vi "query_cmd_single.vi"(6 "Parameter":variant, 7 "Command group":T3(ring), 8 "error in (no error)":errorcluster, 9 "Command ID":u8, 10 "Command subgroup":T2(ring), 11 "VISA resource name":refnum<visa-resource-name>) -> (0 "error out":errorcluster, 1 "formatted response":string, 2 "command packet":string, 3 "VISA resource name out":refnum<visa-resource-name>, 4 "response packet cluster":T1)   [LabVIEW 2018]
doc: "Query a command supported by the IC6 and format the response accordingly."
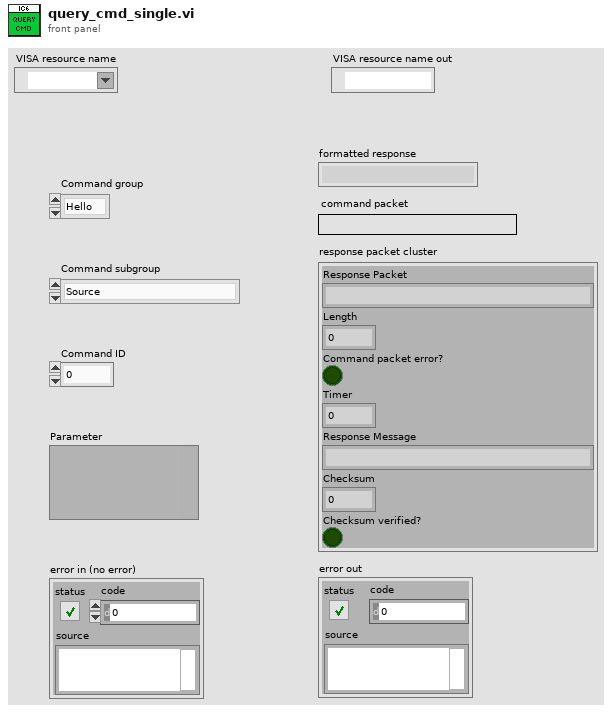
[diagram p1: front panel]
types:
  T1 = cluster{"Response Packet":string, "Length":u16, "Command packet error?":bool, "Timer":u8, "Response Message":string, "Checksum":u8, "Checksum verified?":bool}
  T2 = enum16{"Source", "General", "Input name", "Process name", "Logic", "Material", "Material name", "Output name", "Process", "Sensor", "Output type", "User message", "Layer", ""}
  T3 = enum16{"Hello", "Query", "Remote action", "Status", "Update"}
  T4 = enum16{"big-endian, network order", "native, host order", "little-endian"}
  T5 = enum16{"Crystal Fail", "Max Power", "Test", "A TEST", "R Lock", "L Lock", "Min Power", "Crystal Switch", "Crystal Sw Fail", "Carousel Open", "Control Delay", "Transfer Delay", "RateWatcher Delay", "RateWatcher Hold", "RateWatcher Sample", "Soak Hold Pre Con", "Soak Hold 1", "Soak Hold 2", "Abbr Average", "No or Neg. Average", "Time Pwr Complete", "Clock Hold", "End of Process", "CoDep Not Calibr", "One Layer Tagged", "Layers Tagged", "Too Many Layers", "Source Conflict", "Recorder Conflict", "Unable to Auto-Z", "DAC Error", "Testing XIU", "Backup Sensor", "Backup Delay"}
  T6 = cluster{"statement #":u8, "statement (hex string)":string}
  T7 = cluster{"Process number":u8, "Layer number":u8, "Parameter":i32}
  T8 = cluster{"Process number":u8, "Layer number":u8, "Parameter":dbl}
  T9 = cluster{"Process number":u8, "Layer number":u8, "Parameter":bool}
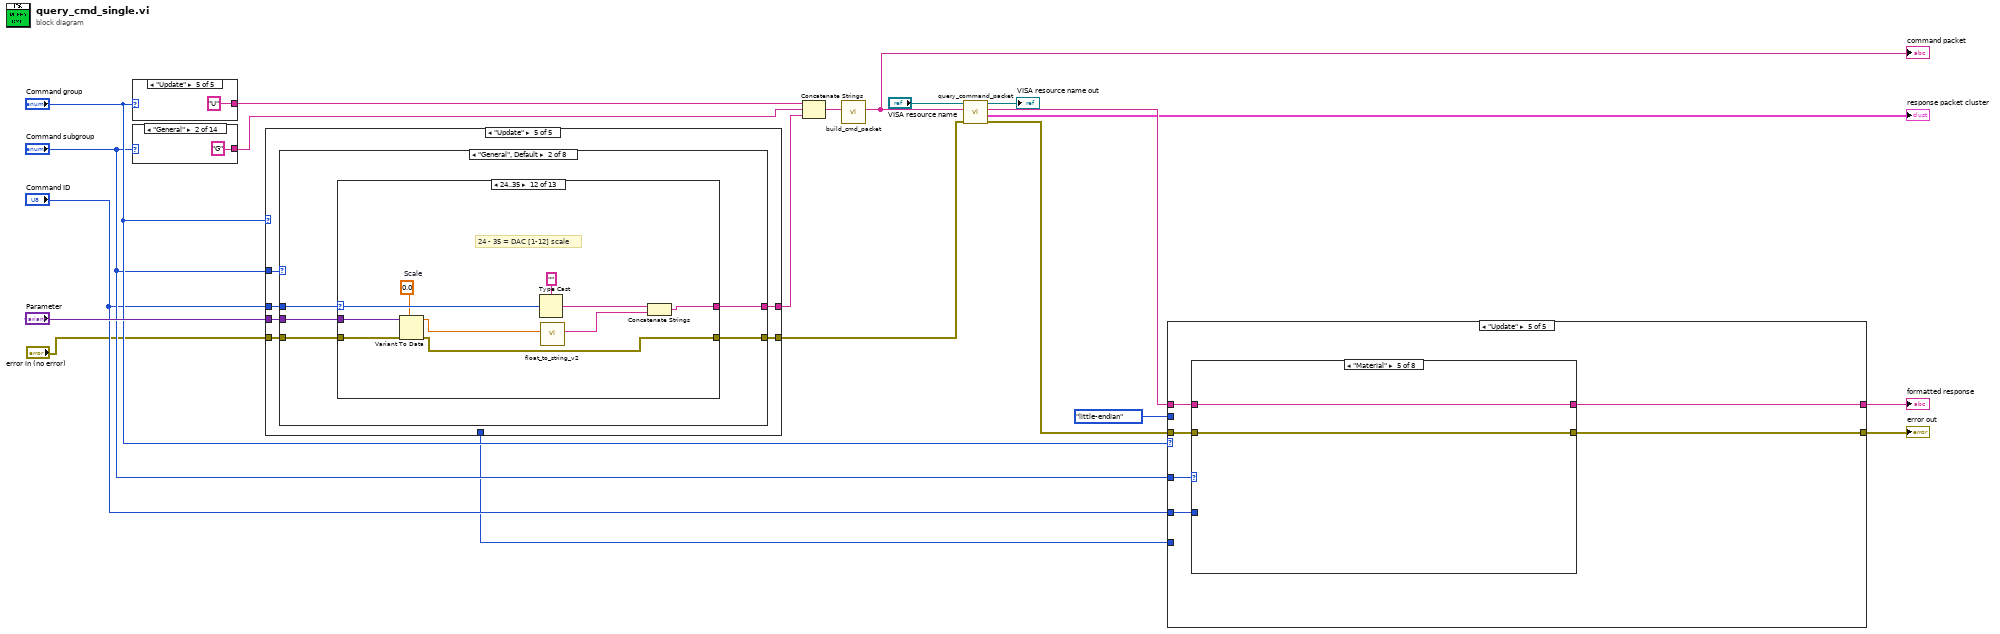
[diagram p0: block diagram]
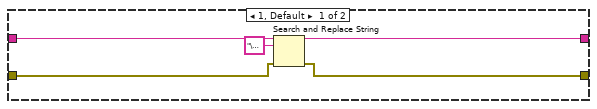
[diagram p3: hidden frame]
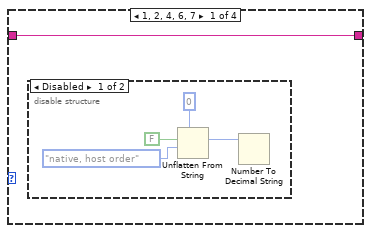
[diagram p6: hidden frame]
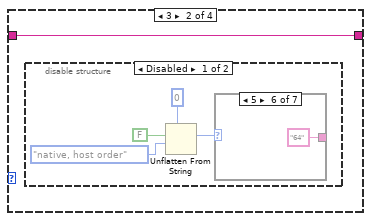
[diagram p8: hidden frame]
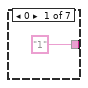
[diagram p9: hidden frame]
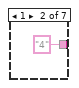
[diagram p10: hidden frame]
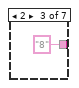
[diagram p11: hidden frame]
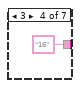
[diagram p12: hidden frame]
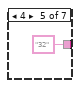
[diagram p13: hidden frame]
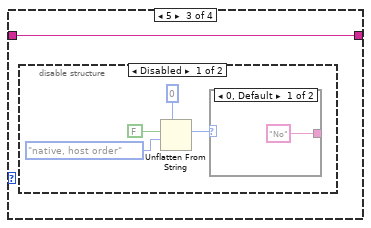
[diagram p16: hidden frame]
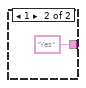
[diagram p17: hidden frame]
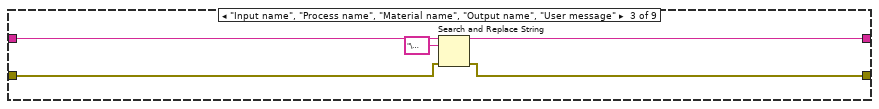
[diagram p20: hidden frame]
diagram:
  n1 = case shown="\"Update\"" "Command group" {
    tunnel: ["H" "Q" "R" "S" "U"] -> w12
    frame "Hello" {
    }
    frame "Query" {
    }
    frame "Remote action" {
    }
    frame "Status" {
    }
    frame "Update" {
    }
  }
  n2 = case shown="\"General\"" "Command subgroup" {
    tunnel: ["C" "G" "I" "K" "L" "M" "N" "O" "P" "S" "T" "V" "L" ""] -> w11
    frame "Source" {
    }
    frame "General" {
    }
    frame "Input name" {
    }
    frame "Process name" {
    }
    frame "Logic" {
    }
    frame "Material" {
    }
    frame "Material name" {
    }
    frame "Output name" {
    }
    frame "Process" {
    }
    frame "Sensor" {
    }
    frame "Output type" {
    }
    frame "User message" {
    }
    frame "Layer" {
    }
    frame "" {
    }
  }
  n3 = case shown="\"Update\"" "Command group" {
    tunnel: "Command subgroup" -> [_ w49 w121 w189 w297]
    tunnel: "Command ID" -> [w43 w48 w119 w188 w300]
    tunnel: "Parameter" -> [_ w47 w120 w186 w299]
    tunnel: [w42 w46 w118 w187 w298] -> w10
    tunnel: [_ _ _ w185 _] -> w15
    tunnel: "error in (no error)" -> [w40 w44 w117 w183 w296]
    tunnel: [w40 w45 w116 w184 w295] -> w3
    frame "Hello" {
      n4 = Type Cast(type="", x=w43) -> (*(type *) &x=w42:string)
    }
    frame "Query" {
      n5 = case shown="\"Source\", Default" w49 {
        tunnel: w48 -> [w55 w64 _ _ w89 w100 w108]
        tunnel: w47 -> [w60 _ w71 w78 w86 w93 w109]
        tunnel: [w56 w63 w70 w74 w81 w92 w107] -> w46
        tunnel: [w50 w61 w65 w72 w79 w90 w105] -> w45
        tunnel: w44 -> [w51 w61 w66 w73 w80 w91 w106]
        frame "Source", Default {
          w54 = u8 0  # Source number
          n6 = Variant To Data(error in=w51, type=w54, Variant=w60) -> (data=w52:u8, error out=w50:errorcluster)
          n7 = Type Cast(type="", x=w55) -> (*(type *) &x=w58:string)
          n8 = Type Cast(type="", x=w52) -> (*(type *) &x=w57:string)
          n9 = Concatenate Strings(w58, w57) -> (w56:string)
        }
        frame "General" {
          n10 = Type Cast(type="", x=w64) -> (*(type *) &x=w63:string)
        }
        frame "Input name", "Process name", "Material name", "Output name", "Output type", "User message" {
          w69 = u8 0  # Number
          n11 = Variant To Data(error in=w66, type=w69, Variant=w71) -> (data=w67:u8, error out=w65:errorcluster)
          n12 = Type Cast(type="", x=w67) -> (*(type *) &x=w70:string)
        }
        frame "Logic" {
          w77 = u8 0  # statement number
          n13 = Variant To Data(error in=w73, type=w77, Variant=w78) -> (data=w75:u8, error out=w72:errorcluster)
          n14 = Type Cast(type="", x=w75) -> (*(type *) &x=w74:string)
        }
        frame "Material" {
          n15 = Variant To Data(error in=w80, type=u8 0, Variant=w86) -> (data=w84:u8, error out=w79:errorcluster)
          n16 = Type Cast(type="", x=w89) -> (*(type *) &x=w83:string)
          n17 = Type Cast(type="", x=w84) -> (*(type *) &x=w82:string)
          n18 = Concatenate Strings(w83, w82) -> (w81:string)
        }
        frame "Process" {
          n19 = Variant To Data(error in=w91, type=cluster{"Process number":u8, "Layer number":u8} {"Process number"=0, "Layer number"=0}, Variant=w93) -> (data=w96:cluster{"Process number":u8, "Layer number":u8}, error out=w90:errorcluster)
          n20 = Unbundle By Name(w96) -> ("Process number"=w95:u8, "Layer number"=w94:u8)
          n21 = Type Cast(type="", x=w94) -> (*(type *) &x=w97:string)
          n22 = Type Cast(type="", x=w100) -> (*(type *) &x=w102:string)
          n23 = Type Cast(type="", x=w95) -> (*(type *) &x=w101:string)
          n24 = Concatenate Strings(w102, w101, w97) -> (w92:string)
        }
        frame "Sensor" {
          w112 = u8 0  # Sensor number
          n25 = Variant To Data(error in=w106, type=w112, Variant=w109) -> (data=w110:u8, error out=w105:errorcluster)
          n26 = Type Cast(type="", x=w108) -> (*(type *) &x=w114:string)
          n27 = Type Cast(type="", x=w110) -> (*(type *) &x=w113:string)
          n28 = Concatenate Strings(w114, w113) -> (w107:string)
        }
      }
    }
    frame "Remote action" {
      n29 = case shown="\"General\", Default" w121 {
        tunnel: w119 -> [w126 w157]
        tunnel: w120 -> [w124 w156]
        tunnel: [w125 w155] -> w118
        tunnel: w117 -> [w122 w154]
        tunnel: [w123 w153] -> w116
        frame "General", Default {
          n30 = case shown="7, 8" w126 {
            selector: w126 -> [w129 w135 w144]
            tunnel: [w128 w133 w146] -> w125
            tunnel: w124 -> [_ w138 w149]
            tunnel: [w127 w131 w142] -> w123
            tunnel: w122 -> [w127 w132 w143]
            frame 0..4, Default {
              # "0=start, 1=stop, 2=reset, 3=remote lock on,\n4=remote lock off"
              n31 = Type Cast(type="", x=w129) -> (*(type *) &x=w128:string)
            }
            frame 5, 6 {
              w139 = u8 0  # Logic statement number
              # "5=set logic statement, 6=clear logic statement"
              n32 = Variant To Data(error in=w132, type=w139, Variant=w138) -> (data=w141:u8, error out=w131:errorcluster)
              n33 = Type Cast(type="", x=w141) -> (*(type *) &x=w134:string)
              n34 = Type Cast(type="", x=w135) -> (*(type *) &x=w137:string)
              n35 = Concatenate Strings(w137, w134) -> (w133:string)
            }
            frame 7, 8 {
              w150 = u8 0  # xtal
              # "7=crystal fail inhibit On (\"Crystal Fail\" outputs always set to False even during crystal fail.),\n8=crystal fail inhibit off (outputs have normal meaning)."
              n36 = Variant To Data(error in=w143, type=w150, Variant=w149) -> (data=w152:u8, error out=w142:errorcluster)
              n37 = Type Cast(type="", x=w152) -> (*(type *) &x=w145:string)
              n38 = Type Cast(type="", x=w144) -> (*(type *) &x=w148:string)
              n39 = Concatenate Strings(w148, w145) -> (w146:string)
            }
          }
        }
        frame "Layer" {
          n40 = case shown="0..6, 8, 9, Default" w157 {
            selector: w157 -> [w162 w179]
            tunnel: w156 -> [w168 w182]
            tunnel: [w161 w178] -> w155
            tunnel: w154 -> [w159 w170]
            tunnel: [w158 w169] -> w153
            frame 0..6, 8, 9, Default {
              w167 = u8 0  # Layer number
              # "0 = suspend, 1 = zero thickness, 2 = start deposit, 3 = go to non-deposit control,\n4 = go to post-deposit, 5 = continue deposit, 6 = go to manual, 8 = open src shutter,\n9 = Close src shutter"
              n41 = Variant To Data(error in=w159, type=w167, Variant=w168) -> (data=w166:u8, error out=w158:errorcluster)
              n42 = Type Cast(type="", x=w166) -> (*(type *) &x=w160:string)
              n43 = Type Cast(type="", x=w162) -> (*(type *) &x=w164:string)
              n44 = Concatenate Strings(w164, w160) -> (w161:string)
            }
            frame 7 {
              # "0 = suspend, 1 = zero thickness, 2 = start deposit, 3 = go to non-deposit control,\n4 = go to post-deposit, 5 = continue deposit, 6 = go to manual"
              n45 = Variant To Data(error in=w170, type=cluster{"Layer number":u8, "Power (%)":sgl} {"Layer number"=0, "Power (%)"=0.0}, Variant=w182) -> (data=w176:cluster{"Layer number":u8, "Power (%)":sgl}, error out=w169:errorcluster)
              n46 = Unbundle(w176) -> ("Layer number"=w174:u8, "Power (%)"=w172:sgl)
              n47 = Type Cast(type="", x=w179) -> (*(type *) &x=w181:string)
              n48 = Type Cast(type="", x=w174) -> (*(type *) &x=w173:string)
              n49 = call "float_to_string_v2.vi"("Float"=w172) -> ("String"=w171:string)  [unwired: 10 in]
              n50 = Concatenate Strings(w181, w173, w171) -> (w178:string)
            }
          }
        }
      }
    }
    frame "Status" {
      n51 = case shown="\"Sensor\"" w189 {
        tunnel: w188 -> [w195 w260 w278]
        tunnel: [w194 w259 w276] -> w187
        tunnel: w186 -> [w193 w261 w277]
        tunnel: [w192 w258 w275] -> w185
        tunnel: [w191 w256 w274] -> w184
        tunnel: w183 -> [w190 w257 w273]
        frame "General", Default {
          n52 = case shown="1..6, 8..10, 15..17, Default" w195 {
            selector: w195 -> [w198 w203 w249]
            tunnel: [w197 w204 w247] -> w194
            tunnel: w193 -> [_ w210 w254]
            tunnel: [0 ("Number") w208 w252] -> w192
            tunnel: [w196 w201 w245] -> w191
            tunnel: w190 -> [w196 w202 w246]
            frame 1..6, 8..10, 15..17, Default {
              # "1 = Active process, 2 = Active layer(s), 3 = Output status, 4 = Input status,\n5 = Logic statement status, 6 = Status messages, 8 = Cause of Stop,\n9 = Transient Messages, 10 = Sensor Status, 15 = Get date, 16 = Get time,\n17 = System configuration (what boards are present)"
              n53 = Type Cast(type="", x=w198) -> (*(type *) &x=w197:string)
            }
            frame 7 {
              # "Status message designators"
              n54 = Variant To Data(error in=w202, type=T5."Crystal Fail" ("Enum"), Variant=w210) -> (data=w208:T5, error out=w201:errorcluster)
              n55 = case shown="\"Crystal Fail\"" w208 {
                tunnel: ["€\u0000\u0000\u0000\u0000\u0000\u0000\u0000" "@\u0000\u0000\u0000\u0000\u0000\u0000\u0000" " \u0000\u0000\u0000\u0000\u0000\u0000\u0000" "\u0010\u0000\u0000\u0000\u0000\u0000\u0000\u0000" "\b\u0000\u0000\u0000\u0000\u0000\u0000\u0000" "\u0004\u0000\u0000\u0000\u0000\u0000\u0000\u0000" "\u0002\u0000\u0000\u0000\u0000\u0000\u0000\u0000" "\u0001\u0000\u0000\u0000\u0000\u0000\u0000\u0000" "\u0000€\u0000\u0000\u0000\u0000\u0000\u0000" "\u0000@\u0000\u0000\u0000\u0000\u0000\u0000" "\u0000 \u0000\u0000\u0000\u0000\u0000\u0000" "\u0000\u0010\u0000\u0000\u0000\u0000\u0000\u0000" "\u0000\b\u0000\u0000\u0000\u0000\u0000\u0000" "\u0000\u0004\u0000\u0000\u0000\u0000\u0000\u0000" "\u0000\u0002\u0000\u0000\u0000\u0000\u0000\u0000" "\u0000\u0001\u0000\u0000\u0000\u0000\u0000\u0000" "\u0000\u0000€\u0000\u0000\u0000\u0000\u0000" "\u0000\u0000@\u0000\u0000\u0000\u0000\u0000" "\u0000\u0000 \u0000\u0000\u0000\u0000\u0000" "\u0000\u0000\u0010\u0000\u0000\u0000\u0000\u0000" "\u0000\u0000\b\u0000\u0000\u0000\u0000\u0000" "\u0000\u0000\u0004\u0000\u0000\u0000\u0000\u0000" "\u0000\u0000\u0002\u0000\u0000\u0000\u0000\u0000" "\u0000\u0000\u0001\u0000\u0000\u0000\u0000\u0000" "\u0000\u0000\u0000€\u0000\u0000\u0000\u0000" "\u0000\u0000\u0000@\u0000\u0000\u0000\u0000" "\u0000\u0000\u0000 \u0000\u0000\u0000\u0000" "\u0000\u0000\u0000\u0010\u0000\u0000\u0000\u0000" "\u0000\u0000\u0000\b\u0000\u0000\u0000\u0000" "\u0000\u0000\u0000\u0004\u0000\u0000\u0000\u0000" "\u0000\u0000\u0000\u0002\u0000\u0000\u0000\u0000" "\u0000\u0000\u0000\u0001\u0000\u0000\u0000\u0000" "\u0000\u0000\u0000\u0000€\u0000\u0000\u0000" "\u0000\u0000\u0000\u0000@\u0000\u0000\u0000"] -> w205
                frame "Crystal Fail" {
                }
                frame "Max Power" {
                }
                frame "Test" {
                }
                frame "A TEST" {
                }
                frame "R Lock" {
                }
                frame "L Lock" {
                }
                frame "Min Power" {
                }
                frame "Crystal Switch" {
                }
                frame "Crystal Sw Fail" {
                }
                frame "Carousel Open" {
                }
                frame "Control Delay" {
                }
                frame "Transfer Delay" {
                }
                frame "RateWatcher Delay" {
                }
                frame "RateWatcher Hold" {
                }
                frame "RateWatcher Sample" {
                }
                frame "Soak Hold Pre Con" {
                }
                frame "Soak Hold 1" {
                }
                frame "Soak Hold 2" {
                }
                frame "Abbr Average" {
                }
                frame "No or Neg. Average" {
                }
                frame "Time Pwr Complete" {
                }
                frame "Clock Hold" {
                }
                frame "End of Process" {
                }
                frame "CoDep Not Calibr" {
                }
                frame "One Layer Tagged" {
                }
                frame "Layers Tagged" {
                }
                frame "Too Many Layers" {
                }
                frame "Source Conflict" {
                }
                frame "Recorder Conflict" {
                }
                frame "Unable to Auto-Z" {
                }
                frame "DAC Error" {
                }
                frame "Testing XIU" {
                }
                frame "Backup Sensor" {
                }
                frame "Backup Delay" {
                }
              }
              n56 = Type Cast(type="", x=w203) -> (*(type *) &x=w207:string)
              n57 = Concatenate Strings(w207, w205) -> (w204:string)
            }
            frame 11..14, 18 {
              w255 = 0  # Number
              # "11 = Timer status, 12 = Timer value,\n13 = Counter value, 14 = Thickness sum,\n18 = Number of layers in process"
              n58 = Variant To Data(error in=w246, type=w255, Variant=w254) -> (data=w252:i32, error out=w245:errorcluster)
              n59 = Type Cast(type="", x=w252) -> (*(type *) &x=w248:string)
              n60 = Type Cast(type="", x=w249) -> (*(type *) &x=w251:string)
              n61 = Concatenate Strings(w251, w248) -> (w247:string)
            }
          }
        }
        frame "Layer" {
          n62 = case shown="1..17, Default" w260 {
            selector: w260 -> [w267]
            tunnel: w261 -> [w272]
            tunnel: [w264] -> w259
            tunnel: [w269] -> w258
            tunnel: w257 -> [w263]
            tunnel: [w262] -> w256
            frame 1..17, Default {
              w271 = u8 0  # Layer
              # "1 = Filtered rate, 2 = Displayed rate, 3 = Source power output, 4 = Thickness, 5 = State, 6 = State time,\n7 = Active sensors, 8 = Power source number, 9 = Accumulated layer time, 10 = Deposit average rate, 11 = Deposit average power, 12 = Raw rate, 13 = One minute averages for rate and power,\n14  = Rate deviation/power output trend, 15 = State before suspend, 16 = Data log,\n17 = Data log with Xtal history"
              n63 = Variant To Data(error in=w263, type=w271, Variant=w272) -> (data=w269:u8, error out=w262:errorcluster)
              n64 = Type Cast(type="", x=w267) -> (*(type *) &x=w266:string)
              n65 = Type Cast(type="", x=w269) -> (*(type *) &x=w265:string)
              n66 = Concatenate Strings(w266, w265) -> (w264:string)
            }
          }
        }
        frame "Sensor" {
          n67 = case shown="0..10, 12, 13, Default" w278 {
            selector: w278 -> [w284 w292]
            tunnel: w277 -> [w287 _]
            tunnel: [w281 w291] -> w276
            tunnel: [w286 u8 0 ("Sensor")] -> w275
            tunnel: [w279 w290] -> w274
            tunnel: w273 -> [w280 w290]
            frame 0..10, 12, 13, Default {
              w289 = u8 0  # Sensor
              # "0 = Crystal life, 1 = Crystals remaining, 2 = Crystal position, 3 = Sensor status,\n4 = Fundamental frequency, 5 = Fundamental Activity, 6 = Current Z-ratio,\n7 = Anharmonic frequency, 8 = Anharmonic activity, 9 = New crystal frequency, 10 = LCQ value,\n12 = Sensor thickness, 13 = Sensor raw rate"
              n68 = Variant To Data(error in=w280, type=w289, Variant=w287) -> (data=w286:u8, error out=w279:errorcluster)
              n69 = Type Cast(type="", x=w284) -> (*(type *) &x=w283:string)
              n70 = Type Cast(type="", x=w286) -> (*(type *) &x=w282:string)
              n71 = Concatenate Strings(w283, w282) -> (w281:string)
            }
            frame 11 {
              # "Not used"
              n72 = Type Cast(type="", x=w292) -> (*(type *) &x=w291:string)
            }
          }
        }
      }
    }
    frame "Update" {
      n73 = case shown="\"General\", Default" w297 {
        tunnel: w300 -> [w305 w346 _ _ w537 w593 w657 _]
        tunnel: w299 -> [w304 w345 w519 w528 w536 w592 w656 w722]
        tunnel: [w303 w344 w518 w522 w531 w591 w652 w718] -> w298
        tunnel: w296 -> [w302 w343 w510 w520 w530 w590 w650 w717]
        tunnel: [w301 w342 w509 w520 w529 w589 w649 w716] -> w295
        frame "Source" {
          n74 = case shown="1..4, 6, 7, Default" w305 {
            selector: w305 -> [w313 w331]
            tunnel: w304 -> [w323 w341]
            tunnel: [w311 w329] -> w303
            tunnel: w302 -> [w306 w326]
            tunnel: [w307 w324] -> w301
            frame 1..4, 6, 7, Default {
              n75 = Variant To Data(error in=w306, type=cluster{"Source number":u8, "Parameter":i32} {"Source number"=0, "Parameter"=0}, Variant=w323) -> (data=w320:cluster{"Source number":u8, "Parameter":i32}, error out=w308:errorcluster)
              n76 = Unbundle(w320) -> ("Source number"=w319:u8, "Parameter"=w310:i32)
              n77 = call "integer_to_string.vi"("error in (no error)"=w308, "number"=w310) -> ("error out"=w307:errorcluster, "String"=w309:string)  [unwired: 8 in]
              n78 = Type Cast(type="", x=w309) -> (*(type *) &x=w316:string)
              n79 = Type Cast(type="", x=w319) -> (*(type *) &x=w317:string)
              n80 = Type Cast(type="", x=w313) -> (*(type *) &x=w315:string)
              n81 = Concatenate Strings(w317, w316) -> (w312:string)
              n82 = Concatenate Strings(w315, w312) -> (w311:string)
            }
            frame 5 {
              n83 = Variant To Data(error in=w326, type=cluster{"Source number":u8, "Parameter":bool} {"Source number"=0, "Parameter"=FALSE}, Variant=w341) -> (data=w338:cluster{"Source number":u8, "Parameter":bool}, error out=w325:errorcluster)
              n84 = Unbundle(w338) -> ("Source number"=w337:u8, "Parameter"=w328:bool)
              n85 = call "boolean_to_string.vi"("error in (no error)"=w325, "Boolean"=w328) -> ("error out"=w324:errorcluster, "String"=w327:string)  [unwired: 8 in]
              n86 = Type Cast(type="", x=w327) -> (*(type *) &x=w334:string)
              n87 = Type Cast(type="", x=w337) -> (*(type *) &x=w336:string)
              n88 = Type Cast(type="", x=w331) -> (*(type *) &x=w333:string)
              n89 = Concatenate Strings(w336, w334) -> (w330:string)
              n90 = Concatenate Strings(w333, w330) -> (w329:string)
            }
          }
        }
        frame "General", Default {
          n91 = case shown="24..35" w346 {
            selector: w346 -> [w349 w357 w370 w380 w390 w399 w412 w428 w443 w457 w476 w492 w503]
            tunnel: w345 -> [_ w361 w372 w382 _ w401 w415 w430 w445 w461 w478 w488 w505]
            tunnel: [w348 w359 w368 w379 w389 w398 w414 w427 w442 w459 w475 w489 w501] -> w344
            tunnel: w343 -> [w347 w354 w365 w376 w388 w395 w409 w424 w439 w455 w472 w485 w498]
            tunnel: [w347 w352 w363 w374 w388 w393 w407 w422 w437 w453 w470 w484 w494] -> w342
            frame 0, Default {
              n92 = Type Cast(type="", x=w349) -> (*(type *) &x=w348:string)
            }
            frame 1..3, 5, 8..11, 16 {
              # "1 = Active process, 2 = Layer to start, 3 = Run number, 5 = Max concurrent layers,\n8 = Active layer output, 9 = Thickness Eq 1, 10 = Thickness Eq 2,\n11 = Thickness Eq 3, 16 = LCD dimmer time (minutes)"
              n93 = Variant To Data(error in=w354, type=0, Variant=w361) -> (data=w355:i32, error out=w353:errorcluster)
              n94 = Type Cast(type="", x=w357) -> (*(type *) &x=w356:string)
              n95 = call "integer_to_string.vi"("error in (no error)"=w353, "number"=w355) -> ("error out"=w352:errorcluster, "String"=w351:string)  [unwired: 8 in]
              n96 = Concatenate Strings(w356, w351) -> (w359:string)
            }
            frame 4, 12..15, 19, 48 {
              w367 = FALSE  # Parameter
              # "12 = Test, 14 = Advanced test (crystal fails active)"
              # "4 = Auto start next, 13 = Time compressed (10x time acceleration), 15 = Audio Feedback,\n19 = Datalog Xtal Info, 48 = Source DAC required"
              n97 = Variant To Data(error in=w365, type=w367, Variant=w372) -> (data=w366:bool, error out=w364:errorcluster)
              n98 = call "boolean_to_string.vi"("error in (no error)"=w364, "Boolean"=w366) -> ("error out"=w363:errorcluster, "String"=w362:string)  [unwired: 8 in]
              n99 = Type Cast(type="", x=w370) -> (*(type *) &x=w369:string)
              n100 = Concatenate Strings(w369, w362) -> (w368:string)
            }
            frame 6 {
              # "Layers displayed"
              n101 = Variant To Data(error in=w376, type="", Variant=w382) -> (data=w383:string, error out=w375:errorcluster)
              n102 = case shown="\"Auto\", Default" w383 {
                tunnel: [0 1 2] -> w377
                frame "Auto", Default {
                }
                frame "4 Layers" {
                }
                frame "6 Layers" {
                }
              }
              n103 = call "integer_to_string.vi"("error in (no error)"=w375, "number"=w377) -> ("error out"=w374:errorcluster, "String"=w373:string)  [unwired: 8 in]
              n104 = Type Cast(type="", x=w380) -> (*(type *) &x=w378:string)
              n105 = Concatenate Strings(w378, w373) -> (w379:string)
            }
            frame 7 {
              # "Not Used"
              n106 = Type Cast(type="", x=w390) -> (*(type *) &x=w389:string)
            }
            frame 17 {
              # "Date format"
              n107 = Variant To Data(error in=w395, type="", Variant=w401) -> (data=w402:string, error out=w394:errorcluster)
              n108 = case shown="\"dd/mm/yyyy\"" w402 {
                tunnel: [0 1] -> w396
                frame "mm/dd/yyyy", Default {
                }
                frame "dd/mm/yyyy" {
                }
              }
              n109 = call "integer_to_string.vi"("error in (no error)"=w394, "number"=w396) -> ("error out"=w393:errorcluster, "String"=w392:string)  [unwired: 8 in]
              n110 = Type Cast(type="", x=w399) -> (*(type *) &x=w397:string)
              n111 = Concatenate Strings(w397, w392) -> (w398:string)
            }
            frame 18 {
              # "USB datalog format"
              n112 = Variant To Data(error in=w409, type="", Variant=w415) -> (data=w416:string, error out=w408:errorcluster)
              n113 = case shown="\"Page\"" w416 {
                tunnel: [0 1 2] -> w410
                frame "Log Off", Default {
                }
                frame "Page" {
                }
                frame "Comma" {
                }
              }
              n114 = call "integer_to_string.vi"("error in (no error)"=w408, "number"=w410) -> ("error out"=w407:errorcluster, "String"=w406:string)  [unwired: 8 in]
              n115 = Type Cast(type="", x=w412) -> (*(type *) &x=w411:string)
              n116 = Concatenate Strings(w411, w406) -> (w414:string)
            }
            frame 20 {
              # "Graph scale"
              n117 = Variant To Data(error in=w424, type="", Variant=w430) -> (data=w431:string, error out=w423:errorcluster)
              n118 = case shown="\"Power\", Default" w431 {
                tunnel: [0 1 2] -> w425
                frame "Power", Default {
                }
                frame "+/-10A/s" {
                }
                frame "+/-20A/s" {
                }
              }
              n119 = call "integer_to_string.vi"("error in (no error)"=w423, "number"=w425) -> ("error out"=w422:errorcluster, "String"=w421:string)  [unwired: 8 in]
              n120 = Type Cast(type="", x=w428) -> (*(type *) &x=w426:string)
              n121 = Concatenate Strings(w426, w421) -> (w427:string)
            }
            frame 21 {
              # "Graph scan rate"
              n122 = Variant To Data(error in=w439, type="", Variant=w445) -> (data=w446:string, error out=w438:errorcluster)
              n123 = case shown="\"Auto\", Default" w446 {
                tunnel: [0 1 2 3] -> w440
                frame "Auto", Default {
                }
                frame "Slow" {
                }
                frame "Med" {
                }
                frame "Fast" {
                }
              }
              n124 = call "integer_to_string.vi"("error in (no error)"=w438, "number"=w440) -> ("error out"=w437:errorcluster, "String"=w436:string)  [unwired: 8 in]
              n125 = Type Cast(type="", x=w443) -> (*(type *) &x=w441:string)
              n126 = Concatenate Strings(w441, w436) -> (w442:string)
            }
            frame 22 {
              # "RS-232 Baud Rate"
              n127 = Variant To Data(error in=w455, type="", Variant=w461) -> (data=w462:string, error out=w454:errorcluster)
              n128 = case shown="\"9600\", Default" w462 {
                tunnel: [0 1 2 3 4] -> w456
                frame "9600", Default {
                }
                frame "19200" {
                }
                frame "38400" {
                }
                frame "57600" {
                }
                frame "115200" {
                }
              }
              n129 = call "integer_to_string.vi"("error in (no error)"=w454, "number"=w456) -> ("error out"=w453:errorcluster, "String"=w452:string)  [unwired: 8 in]
              n130 = Type Cast(type="", x=w457) -> (*(type *) &x=w458:string)
              n131 = Concatenate Strings(w458, w452) -> (w459:string)
            }
            frame 23 {
              # "RS-232 protocol"
              n132 = Variant To Data(error in=w472, type="", Variant=w478) -> (data=w479:string, error out=w471:errorcluster)
              n133 = case shown="\"Standard\", Default" w479 {
                tunnel: [0 1 2] -> w473
                frame "Standard", Default {
                }
                frame "Dlog Comma" {
                }
                frame "Dlog Page" {
                }
              }
              n134 = call "integer_to_string.vi"("error in (no error)"=w471, "number"=w473) -> ("error out"=w470:errorcluster, "String"=w469:string)  [unwired: 8 in]
              n135 = Type Cast(type="", x=w476) -> (*(type *) &x=w474:string)
              n136 = Concatenate Strings(w474, w469) -> (w475:string)
            }
            frame 24..35 {
              w487 = sgl 0.0  # Scale
              # "24 - 35 = DAC [1-12] scale"
              n137 = Variant To Data(error in=w485, type=w487, Variant=w488) -> (data=w486:sgl, error out=w484:errorcluster)
              n138 = Type Cast(type="", x=w492) -> (*(type *) &x=w491:string)
              n139 = call "float_to_string_v2.vi"("Float"=w486) -> ("String"=w490:string)  [unwired: 10 in]
              n140 = Concatenate Strings(w491, w490) -> (w489:string)
            }
            frame 36..47 {
              # "36 - 47 = DAC [1-12] polarity"
              n141 = Variant To Data(error in=w498, type="", Variant=w505) -> (data=w500:string, error out=w497:errorcluster)
              n142 = To Lower Case(string=w500) -> (all lower case string=w499:string)
              n143 = case shown="\"positive\", Default" w499 {
                tunnel: [u8 0 u8 1] -> w496
                frame "negative" {
                }
                frame "positive", Default {
                }
              }
              n144 = call "integer_to_string.vi"("error in (no error)"=w497, "number"=w496) -> ("error out"=w494:errorcluster, "String"=w495:string)  [unwired: 8 in]
              n145 = Type Cast(type="", x=w503) -> (*(type *) &x=w502:string)
              n146 = Concatenate Strings(w502, w495) -> (w501:string)
            }
          }
        }
        frame "Input name", "Process name", "Material name", "Output name", "User message" {
          n147 = Variant To Data(error in=w510, type=cluster{"Number":u8, "Name":string} {"Number"=0, "Name"=""}, Variant=w519) -> (data=w515:cluster{"Number":u8, "Name":string}, error out=w509:errorcluster)
          n148 = Unbundle(w515) -> ("Number"=w514:u8, "Name"=w512:string)
          n149 = Type Cast(type="", x=w514) -> (*(type *) &x=w513:string)
          n150 = Concatenate Strings(w513, w512, "\u0000" ("string")) -> (w518:string)
        }
        frame "Logic" {
          n151 = Variant To Data(type=T6 {"statement #"=0, "statement (hex string)"=""}, Variant=w528) -> (data=w526:T6)  [unwired: 1 in, 1 out]
          n152 = Unbundle(w526) -> ("statement #"=w524:u8, "statement (hex string)"=w521:string)
          n153 = Type Cast(type="", x=w524) -> (*(type *) &x=w523:string)
          n154 = Concatenate Strings(w523, w521) -> (w522:string)
        }
        frame "Material" {
          n155 = case shown="1..3, 5..7, 9, 10, 12, 15, 18, 27, 28, 31, 33, 39, 40, 42, 43, 66..97, 116, 120" w537 {
            selector: w537 -> [w539 w545 w557 w569 w581]
            tunnel: ["" w546 w558 w570 w582] -> w532
            tunnel: w536 -> [_ w547 w559 w571 w583]
            tunnel: [w539 w545 w557 w569 w581] -> w533
            tunnel: w530 -> [w538 w542 w554 w566 w578]
            tunnel: [w538 w541 w553 w565 w577] -> w529
            frame 0, Default {
            }
            frame 1..3, 5..7, 9, 10, 12, 15, 18, 27, 28, 31, 33, 39, 40, 42, 43, 66..97, 116, 120 {
              # "1 = Density (g/cc), 2 = Z-ratio, 3=Master tooling (%), 5=Process Gain (A/s/%), 6=Time\nConstant (s), 7=Dead time (seconds), 9=Maximum power (%), 10=Minimum power (%), 12=\nPreCond Soak Power (%), 15=Soak power 1 (%), 18= Soak power 2 (%), 27=Transfer tooling\n(%), 28=Feed power (%), 31=Idle power (%), 33=Rate (A/s), 39=Ramp 1 rate (A/s), 40=Start\nramp 1 (kA), 42=Ramp 2 rate (A/s), 43= Start ramp 2 (kA), 66-73=Sensor [1-8] Weight (%),\n74-81=Sensor [1-8] Tooling (%), 82-89=Sensor [1-8] CrystalTwo Tooling (%), 90-97=Sensor\n[1-8] cal thickness (kA), 116=CrystalTwo Tooling (%), 120=Backup Tooling (%)"
              n156 = Variant To Data(error in=w542, type=cluster{"Material number":u8, "Parameter":sgl} {"Material number"=0, "Parameter"=0.0}, Variant=w547) -> (data=w550:cluster{"Material number":u8, "Parameter":sgl}, error out=w541:errorcluster)
              n157 = Unbundle(w550) -> ("Material number"=w551:u8, "Parameter"=w544:sgl)
              n158 = Type Cast(type="", x=w551) -> (*(type *) &x=w552:string)
              n159 = call "float_to_string_v2.vi"("Float"=w544) -> ("String"=w543:string)  [unwired: 10 in]
              n160 = Concatenate Strings(w552, w543) -> (w546:string)
            }
            frame 4, 8, 11, 23, 25, 26, 35, 36, 38, 47, 50..65, 98..115, 117..119, 121..127 {
              # "4=Control Loop, 8=Source, 11=Max Power Option, 23=Delay Option, 25=Shutter delay accur\n(%), 26=Transfer Sensor, 35=Rate filter time (s), 36=Time Pow Avg (mins), 38=On final\nthickness, 47=RateWatcher Accuracy,\n50-57=Sensor [1-8] Failure Action, 58-65=Sensor [1-8] Failure Trigger, 98-105=Sensor [1-8]\nXtal position first, 106-113=Sensor [1-8] Xtal position last, 114=Sensor, 115=Failure action,\n117=Xtal position first, 118=Xtal position last, 119=Backup sensor, 121=Quality percent (%)\n122=Quality counts, 123=Stability single (Hz), 124=Stability total (Hz), 125=Recorder output\n126=Recorder function, 127=Recorder range"
              n161 = Variant To Data(error in=w554, type=cluster{"Material number":u8, "Parameter":i32} {"Material number"=0, "Parameter"=0}, Variant=w559) -> (data=w562:cluster{"Material number":u8, "Parameter":i32}, error out=w553:errorcluster)
              n162 = Unbundle(w562) -> ("Material number"=w563:u8, "Parameter"=w556:i32)
              n163 = call "integer_to_string.vi"("number"=w556) -> ("String"=w555:string)  [unwired: 9 in, 1 out]
              n164 = Type Cast(type="", x=w563) -> (*(type *) &x=w564:string)
              n165 = Concatenate Strings(w564, w555) -> (w558:string)
            }
            frame 13, 14, 16, 17, 19, 20, 24, 29, 30, 32, 34, 41, 44, 46 {
              # "13=PreCond Rise time (s), 14=PreCond soak time (s), 16=Rise time 1 (s), 17=Soak time 1 (s)\n19=Rise time 2 (s), 20=Soak time 2 (s), 24=Control delay time (s), 29=Feed ramp time (s),\n30=Feed time (s), 32=Idle ramp time (s), 34=Time limit (s), 41=Ramp 1 time (s),\n44=Ramp 2 time (s), 46=RateWatcher time (s)"
              n166 = Variant To Data(error in=w566, type=cluster{"Material number":u8, "Parameter":u16} {"Material number"=0, "Parameter"=0}, Variant=w571) -> (data=w574:cluster{"Material number":u8, "Parameter":u16}, error out=w565:errorcluster)
              n167 = Unbundle(w574) -> ("Material number"=w575:u8, "Parameter"=w568:u16)
              n168 = Type Cast(type="", x=w575) -> (*(type *) &x=w576:string)
              n169 = call "integer_to_string.vi"("number"=w568) -> ("String"=w567:string)  [unwired: 9 in, 1 out]
              n170 = Concatenate Strings(w576, w567) -> (w570:string)
            }
            frame 21, 22, 37, 45, 48, 49 {
              # "21=Auto soak 2, 22=Dep after pre-dep, 37=Ion assist deposit, 45=RateWatcher Option\n48=Multipoint, 49=Aggregate multiplier"
              n171 = Variant To Data(error in=w578, type=cluster{"Material number":u8, "State":bool} {"Material number"=0, "State"=FALSE}, Variant=w583) -> (data=w586:cluster{"Material number":u8, "State":bool}, error out=w577:errorcluster)
              n172 = Unbundle(w586) -> ("Material number"=w587:u8, "State"=w580:bool)
              n173 = Type Cast(type="", x=w587) -> (*(type *) &x=w588:string)
              n174 = call "boolean_to_string.vi"("Boolean"=w580) -> ("String"=w579:string)  [unwired: 9 in, 1 out]
              n175 = Concatenate Strings(w588, w579) -> (w582:string)
            }
          }
          n176 = Type Cast(type="", x=w533) -> (*(type *) &x=w535:string)
          n177 = Concatenate Strings(w535, w532) -> (w531:string)
        }
        frame "Process" {
          n178 = case shown="2, 3, 6" w593 {
            selector: w593 -> [_ w605 w623 w640]
            tunnel: w592 -> [_ w613 w630 w647]
            tunnel: [_ w601 w619 w636] -> w591
            tunnel: w590 -> [w594 w597 w616 w633]
            tunnel: [w594 w595 w615 w632] -> w589
            frame 0, Default {
            }
            frame 1, 4 {
              # "1=Material, 4=Cruc"
              n179 = Variant To Data(error in=w597, type=T7 {"Process number"=0, "Layer number"=0, "Parameter"=0}, Variant=w613) -> (data=w604:T7, error out=w596:errorcluster)
              n180 = Unbundle By Name(w604) -> ("Process number"=w603:u8, "Layer number"=w602:u8, "Parameter"=w599:i32)
              n181 = call "integer_to_string.vi"("error in (no error)"=w596, "number"=w599) -> ("error out"=w595:errorcluster, "String"=w598:string)  [unwired: 8 in]
              n182 = Type Cast(type="", x=w598) -> (*(type *) &x=w600:string)
              n183 = Type Cast(type="", x=w602) -> (*(type *) &x=w607:string)
              n184 = Type Cast(type="", x=w605) -> (*(type *) &x=w610:string)
              n185 = Type Cast(type="", x=w603) -> (*(type *) &x=w609:string)
              n186 = Concatenate Strings(w610, w609, w607, w600) -> (w601:string)
            }
            frame 2, 3, 6 {
              # "6=Ratio Cntrl (%)"
              # "2=Final thick, 3=Thick limit"
              n187 = Variant To Data(error in=w616, type=T8 {"Process number"=0, "Layer number"=0, "Parameter"=0.0}, Variant=w630) -> (data=w622:T8, error out=w615:errorcluster)
              n188 = Unbundle By Name(w622) -> ("Process number"=w621:u8, "Layer number"=w620:u8, "Parameter"=w618:dbl)
              n189 = Type Cast(type="", x=w623) -> (*(type *) &x=w627:string)
              n190 = Type Cast(type="", x=w621) -> (*(type *) &x=w626:string)
              n191 = Type Cast(type="", x=w620) -> (*(type *) &x=w624:string)
              n192 = call "float_to_string_v2.vi"("Float"=w618) -> ("String"=w617:string)  [unwired: 10 in]
              n193 = Concatenate Strings(w627, w626, w624, w617) -> (w619:string)
            }
            frame 5 {
              # "5=CoDep"
              n194 = Variant To Data(error in=w633, type=T9 {"Process number"=0, "Layer number"=0, "Parameter"=FALSE}, Variant=w647) -> (data=w639:T9, error out=w632:errorcluster)
              n195 = Unbundle By Name(w639) -> ("Process number"=w638:u8, "Layer number"=w637:u8, "Parameter"=w635:bool)
              n196 = Type Cast(type="", x=w640) -> (*(type *) &x=w644:string)
              n197 = Type Cast(type="", x=w638) -> (*(type *) &x=w643:string)
              n198 = Type Cast(type="", x=w637) -> (*(type *) &x=w641:string)
              n199 = call "boolean_to_string.vi"("Boolean"=w635) -> ("String"=w634:string)  [unwired: 9 in, 1 out]
              n200 = Concatenate Strings(w644, w643, w641, w634) -> (w636:string)
            }
          }
        }
        frame "Sensor" {
          n201 = case shown="0, Default" w657 {
            selector: w657 -> [w659 w666 w681 w695 w708]
            tunnel: w656 -> [_ w675 w690 w702 w715]
            tunnel: ["" w667 w682 w696 w709] -> w653
            tunnel: [w659 w666 w681 w695 w708] -> w654
            tunnel: w650 -> [w658 w663 w678 w692 w705]
            tunnel: [w658 w661 w676 w691 w703] -> w649
            frame 0, Default {
            }
            frame 1..3, 5, 6, 9, 10 {
              # "1=Sensor shutter output, 2=Sensor type, 3=Sensor switch output, 5=# of positions,\n6=# of pulses, 9=Recorder ouptut, 10=Recorder function"
              n202 = Variant To Data(error in=w663, type=cluster{"Sensor number":u8, "Parameter":i32} {"Sensor number"=1, "Parameter"=0}, Variant=w675) -> (data=w672:cluster{"Sensor number":u8, "Parameter":i32}, error out=w662:errorcluster)
              n203 = Unbundle(w672) -> ("Sensor number"=w670:u8, "Parameter"=w665:i32)
              n204 = call "integer_to_string.vi"("error in (no error)"=w662, "number"=w665) -> ("error out"=w661:errorcluster, "String"=w664:string)  [unwired: 8 in]
              n205 = Type Cast(type="", x=w670) -> (*(type *) &x=w669:string)
              n206 = Type Cast(type="", x=w664) -> (*(type *) &x=w668:string)
              n207 = Concatenate Strings(w669, w668) -> (w667:string)
            }
            frame 4 {
              # "Auto-Z"
              n208 = Variant To Data(error in=w678, type=cluster{"Sensor number":u8, "Auto-Z":bool} {"Sensor number"=1, "Auto-Z"=FALSE}, Variant=w690) -> (data=w687:cluster{"Sensor number":u8, "Auto-Z":bool}, error out=w677:errorcluster)
              n209 = Unbundle(w687) -> ("Sensor number"=w685:u8, "Auto-Z"=w680:bool)
              n210 = call "boolean_to_string.vi"("error in (no error)"=w677, "Boolean"=w680) -> ("error out"=w676:errorcluster, "String"=w679:string)  [unwired: 8 in]
              n211 = Type Cast(type="", x=w685) -> (*(type *) &x=w684:string)
              n212 = Type Cast(type="", x=w679) -> (*(type *) &x=w683:string)
              n213 = Concatenate Strings(w684, w683) -> (w682:string)
            }
            frame 7, 8 {
              # "7=Pulse on time (s), 8=Pulse off time (s)"
              n214 = Variant To Data(error in=w692, type=cluster{"Sensor number":u8, "Parameter":sgl} {"Sensor number"=1, "Parameter"=0.0}, Variant=w702) -> (data=w700:cluster{"Sensor number":u8, "Parameter":sgl}, error out=w691:errorcluster)
              n215 = Unbundle(w700) -> ("Sensor number"=w698:u8, "Parameter"=w693:sgl)
              n216 = call "float_to_string_v2.vi"("Float"=w693) -> ("String"=w694:string)  [unwired: 10 in]
              n217 = Type Cast(type="", x=w698) -> (*(type *) &x=w697:string)
              n218 = Concatenate Strings(w697, w694) -> (w696:string)
            }
            frame 11 {
              # "11=Recorder range"
              n219 = Variant To Data(error in=w705, type=cluster{"Sensor number":u8, "Parameter":i32} {"Sensor number"=1, "Parameter"=0}, Variant=w715) -> (data=w713:cluster{"Sensor number":u8, "Parameter":i32}, error out=w704:errorcluster)
              n220 = Unbundle(w713) -> ("Sensor number"=w711:u8, "Parameter"=w707:i32)
              n221 = call "integer_to_string.vi"("error in (no error)"=w704, "number"=w707) -> ("error out"=w703:errorcluster, "String"=w706:string)  [unwired: 8 in]
              n222 = Type Cast(type="", x=w711) -> (*(type *) &x=w710:string)
              n223 = Concatenate Strings(w710, w706) -> (w709:string)
            }
          }
          n224 = Type Cast(type="", x=w654) -> (*(type *) &x=w651:string)
          n225 = Concatenate Strings(w651, w653) -> (w652:string)
        }
        frame "Output type" {
          n226 = Variant To Data(error in=w717, type=cluster{"Number":u8, "Type":u8} {"Number"=0, "Type"=0}, Variant=w722) -> (data=w725:cluster{"Number":u8, "Type":u8}, error out=w716:errorcluster)
          n227 = Unbundle(w725) -> ("Number"=w724:u8, "Type"=w720:u8)
          n228 = Type Cast(type="", x=w720) -> (*(type *) &x=w719:string)
          n229 = Type Cast(type="", x=w724) -> (*(type *) &x=w723:string)
          n230 = Concatenate Strings(w723, w719) -> (w718:string)
        }
      }
    }
  }
  n231 = Concatenate Strings(w12, w11, w10) -> (w13:string)
  n232 = call "build_cmd_packet.vi"("message"=w13) -> ("command packet"=w9:string)  [unwired: 10 in]
  "command packet" <- w9
  n233 = call "query_command_packet.vi"("error in (no error)"=w3, "command packet"=w9, "VISA resource name"="VISA resource name") -> ("error out"=w2:errorcluster, "response packet cluster"=→"response packet cluster":T1, "response"=w8:string, "VISA resource name out"=→"VISA resource name out":refnum<visa-resource-name>)  [unwired: 5 in]
  n234 = case shown="\"Update\"" "Command group" {
    tunnel: "Command subgroup" -> [_ w745 _ w804 w897]
    tunnel: "Command ID" -> [w732 w744 _ w802 w896]
    tunnel: w8 -> [w731 w743 w796 w801 w898]
    tunnel: [w730 w742 w796 w799 w895] -> w17
    tunnel: w15 -> [_ _ _ w803 _]
    tunnel: T4."little-endian" ("byte order (0:big-endian, network order)") -> [_ _ _ w800 _]
    tunnel: w2 -> [w729 w741 w795 w798 w893]
    tunnel: [w728 w740 w795 w797 w894] -> w1
    frame "Hello" {
      n235 = case shown="2, 3" w732 {
        tunnel: [w735 w739] -> w730
        tunnel: w731 -> [w736 w739]
        tunnel: w729 -> [w734 w738]
        tunnel: [w733 w738] -> w728
        frame 1, Default {
          n236 = Search and Replace String(input string=w736, search string="\u0000", error in=w734) -> (result string=w735:string, error out=w733:errorcluster)  [unwired: 5 in, 2 out]
        }
        frame 2, 3 {
        }
      }
    }
    frame "Query" {
      n237 = case shown="\"Process\"" w745 {
        tunnel: w744 -> [w749 _ _ _ _ _ _ _ _]
        tunnel: w743 -> [w748 w775 w779 w782 w786 w788 w790 w792 w794]
        tunnel: [w747 w775 w778 w782 w784 w788 w790 w792 w794] -> w742
        tunnel: w741 -> [w746 w774 w777 w781 w783 w787 w789 w791 w793]
        tunnel: [w746 w774 w776 w781 w783 w787 w789 w791 w793] -> w740
        frame "Source" {
          n238 = case shown="Default" w749 {
            tunnel: w748 -> [w750 w755 w766 w773]
            tunnel: [w750 w755 w766 w773] -> w747
            frame 1, 2, 4, 6, 7 {
              n239 = disable-structure shown="Disabled" {
                frame Disabled {
                  n240 = Unflatten From String(type=0, data includes array or string size? (T)=FALSE, byte order (0:big-endian, network order)=T4."native, host order") -> (value=w751:i32)  [unwired: 2 in, 2 out]
                  n241 = Number To Decimal String(number=w751) -> ()  [unwired: 1 in, 1 out]
                }
                frame Enabled {
                }
              }
            }
            frame 3 {
              n242 = disable-structure shown="Disabled" {
                frame Disabled {
                  n243 = Unflatten From String(type=0, data includes array or string size? (T)=FALSE, byte order (0:big-endian, network order)=T4."native, host order") -> (value=w756:i32)  [unwired: 2 in, 2 out]
                  n244 = case shown="5" w756 {
                    tunnel: ["1" "4" "8" "16" "32" "64" _] -> _
                    frame 0 {
                    }
                    frame 1 {
                    }
                    frame 2 {
                    }
                    frame 3 {
                    }
                    frame 4 {
                    }
                    frame 5 {
                    }
                    frame 6, Default {
                    }
                  }
                }
                frame Enabled {
                }
              }
            }
            frame 5 {
              n245 = disable-structure shown="Disabled" {
                frame Disabled {
                  n246 = Unflatten From String(type=0, data includes array or string size? (T)=FALSE, byte order (0:big-endian, network order)=T4."native, host order") -> (value=w767:i32)  [unwired: 2 in, 2 out]
                  n247 = case shown="0, Default" w767 {
                    tunnel: ["No" "Yes"] -> _
                    frame 0, Default {
                    }
                    frame 1 {
                    }
                  }
                }
                frame Enabled {
                }
              }
            }
            frame Default {
            }
          }
        }
        frame "General" {
        }
        frame "Input name", "Process name", "Material name", "Output name", "User message" {
          n248 = Search and Replace String(input string=w779, search string="\u0000", error in=w777) -> (result string=w778:string, error out=w776:errorcluster)  [unwired: 5 in, 2 out]
        }
        frame "Output type" {
        }
        frame "Logic" {
          n249 = String Subset(string=w786, offset (0)=1) -> (substring=w784:string)  [unwired: 1 in]
        }
        frame "Material" {
        }
        frame "Process" {
        }
        frame "Sensor" {
        }
        frame Default {
        }
      }
    }
    frame "Remote action" {
    }
    frame "Status" {
      n250 = case shown="\"General\", Default" w804 {
        tunnel: w803 -> [_ _ w879]
        tunnel: w802 -> [w810 _ w880]
        tunnel: w801 -> [w809 w873 w878]
        tunnel: w800 -> [w808 _ _]
        tunnel: [w807 w873 w877] -> w799
        tunnel: w798 -> [w806 w874 w875]
        tunnel: [w805 w874 w876] -> w797
        frame "General", Default {
          n251 = case shown="7" w810 {
            tunnel: w809 -> [w818 w830 w838 w839 w842 w850]
            tunnel: w808 -> [w816 _ _ _ _ w848]
            tunnel: [w813 w820 w838 w839 w842 w845] -> w807
            tunnel: w806 -> [w812 w819 w837 w840 w841 w844]
            tunnel: [w811 w819 w837 w840 w841 w843] -> w805
            frame 1, 12, 13, 18, Default {
              n252 = Unflatten From String(type=0, binary string=w818, data includes array or string size? (T)=FALSE, byte order (0:big-endian, network order)=w816, error in (no error)=w812) -> (value=w814:i32, error out=w811:errorcluster)  [unwired: 1 out]
              n253 = Number To Decimal String(number=w814) -> (decimal integer string=w813:string)  [unwired: 1 in]
            }
            frame 2 {
              # "Forms a comma separated string of which layers are active"
              n254 = String To Byte Array(string=w830) -> (unsigned byte array=w828:u8[])
              n255 = Index Array(array=w828, index=0) -> (element=w827:u8)
              n256 = Array Subset(array=w828, index=1, length=w827) -> (w825:u8[])
              n257 = for {
                tunnel: w825 -> [w836] mode=indexing
                shift-right: [w832] -> w823
                shift-left: "" -> [w834]
                n258 = Type Cast(type="", x=w836) -> (*(type *) &x=w833:string)
                n259 = Concatenate Strings(w834, w833, "," ("string")) -> (w832:string)
              }
              n260 = String Length(string=w823) -> (length=w822:i32)
              n261 = Decrement(x=w822) -> (x-1=w821:i32)
              n262 = String Subset(string=w823, length (rest)=w821) -> (substring=w820:string)  [unwired: 1 in]
            }
            frame 3..5 {
            }
            frame 6 {
            }
            frame 7 {
            }
            frame 8 {
              n263 = Unflatten From String(type=u8 0, binary string=w850, data includes array or string size? (T)=FALSE, byte order (0:big-endian, network order)=w848, error in (no error)=w844) -> (value=w846:u8, error out=w843:errorcluster)  [unwired: 1 out]
              n264 = case shown="1, Default" w846 {
                tunnel: ["Max power" "Crystal Fail" "Hand Controller" "Front Panel" "Communication" "Crucible Fail" "Switcher Fail" "Logic Eqn #" "No Source DAC" "Power Loss" "Source Conflict" "Sensor Conflict" "Shutter Fail" "CrossTalk > 100%" "DAC Failure" "Half Rate Fail" "Low Rate" "AutoTune Fail" "Quick Tune Fail" "Bad Co-Dep Load" "Uncalibrated" "Bad Layer Load"] -> w845
                frame 1, Default {
                }
                frame 2 {
                }
                frame 3 {
                }
                frame 4 {
                }
                frame 5 {
                }
                frame 6 {
                }
                frame 7 {
                }
                frame 8 {
                }
                frame 9 {
                }
                frame 10 {
                }
                frame 11 {
                }
                frame 12 {
                }
                frame 13 {
                }
                frame 14 {
                }
                frame 15 {
                }
                frame 16 {
                }
                frame 17 {
                }
                frame 18 {
                }
                frame 19 {
                }
                frame 20 {
                }
                frame 21 {
                }
                frame 22 {
                }
              }
            }
          }
        }
        frame "Layer" {
        }
        frame "Sensor" {
          n265 = case shown="0..3, Default" w880 {
            tunnel: w879 -> [_ _ _ _ _ _]
            tunnel: w878 -> [w882 w884 w886 w888 w890 w892]
            tunnel: [w882 w884 w886 w888 w890 w892] -> w877
            tunnel: [w881 w883 w885 w887 w889 w891] -> w876
            tunnel: w875 -> [w881 w883 w885 w887 w889 w891]
            frame 0..3, Default {
            }
            frame 4, 7 {
            }
            frame 5, 8 {
            }
            frame 6, 10, 12, 13 {
            }
            frame 9 {
              # "Not implemented"
            }
            frame 11 {
              # "Not used"
            }
          }
        }
      }
    }
    frame "Update" {
      n266 = case shown="\"Material\"" w897 {
        tunnel: w896 -> [w903 _ w912 _ _ _ _ _]
        tunnel: w898 -> [w902 w907 w911 w916 w918 w920 w922 w924]
        tunnel: [w901 w907 w910 w916 w918 w920 w922 w924] -> w895
        tunnel: [w900 w906 w909 w915 w917 w919 w921 w923] -> w894
        tunnel: w893 -> [w899 w906 w908 w915 w917 w919 w921 w923]
        frame "Source", Default {
          n267 = case shown="1..7, Default" w903 {
            tunnel: w902 -> [w905]
            tunnel: [w905] -> w901
            tunnel: [w904] -> w900
            tunnel: w899 -> [w904]
            frame 1..7, Default {
            }
          }
        }
        frame "General" {
        }
        frame "Input name", "Process name", "Material name", "Output name", "User message" {
          n268 = case shown="0, Default" w912 {
            tunnel: [w914] -> w910
            tunnel: w911 -> [w914]
            tunnel: [w913] -> w909
            tunnel: w908 -> [w913]
            frame 0, Default {
            }
          }
        }
        frame "Logic" {
        }
        frame "Material" {
        }
        frame "Process" {
        }
        frame "Sensor" {
        }
        frame "Output type" {
        }
      }
    }
  }
  "error out" <- w1
  "formatted response" <- w17
